vi "Importing FFT Data class VI - change data.vi"(6 "FFTs Table":string[][](array[string]), 7 "Row":i32, 8 "error in (no error)":errorcluster, 9 "Array 2":dbl[][](array[numeric]), 10 "Array":dbl[][](array[numeric]), 11 "Imported FFT Data in":refnum<class "Imported FFT Data.lvclass">) -> (0 "error out":errorcluster, 3 "Imported FFT Data out":refnum<class "Imported FFT Data.lvclass">)   [LabVIEW 2010, in "Imported FFT Data.lvclass"]
uses:
  Imported FFT Data.lvclass
  Imported FFT Data.lvclass/Imported FFT Data.ctl
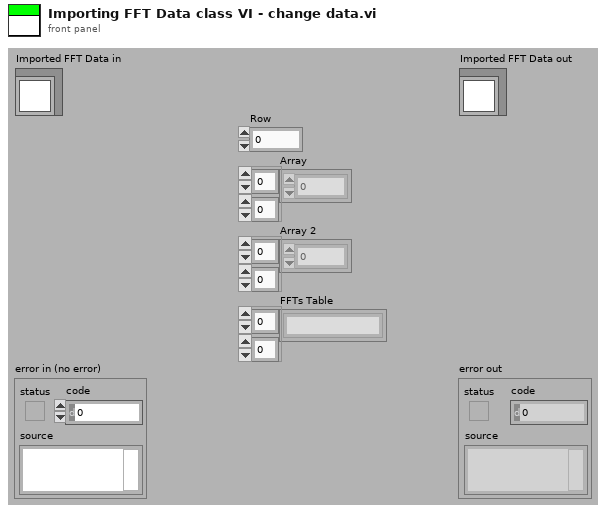
[diagram p1: front panel]
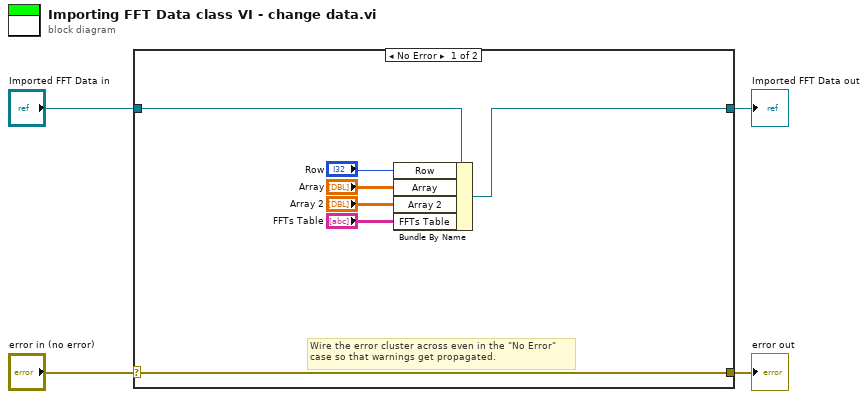
[diagram p0: block diagram]
diagram:
  n1 = case shown="No Error" "error in (no error)" {
    selector: "error in (no error)" -> [w11 w13]
    tunnel: [w11 w13] -> w3
    tunnel: [w9 w12] -> w1
    tunnel: "Imported FFT Data in" -> [w10 w12]
    frame No Error {
      # "Wire the error cluster across even in the \"No Error\"\ncase so that warnings get propagated."
      n2 = Bundle By Name(cluster=w10, "Row"="Row", "Array"="Array", "Array 2"="Array 2", "FFTs Table"="FFTs Table") -> (w9:refnum<class "Imported FFT Data.lvclass">)
    }
    frame Error {
    }
  }
  "error out" <- w3
  "Imported FFT Data out" <- w1
